vi "MatrixTest1.vi"() -> ()   [LabVIEW 2024]
uses:
  <vilib>/Analysis/baseanly.llb/Real A x B.vi
  <vilib>/Analysis/7linalg.llb/Real Transpose Matrix.vi
  <vilib>/Analysis/Matrix/Numeric/Conversions/Array To Matrix - RA.vi
  <vilib>/Analysis/Matrix/Numeric/Conversions/Matrix To Array - RM.vi
  <vilib>/Analysis/NI_AALBase.lvlib
  <vilib>/Analysis/Matrix/NI_Matrix.lvlib
  <vilib>/Analysis/NI_AALPro.lvlib
panel:
  in  "Array 11":i16[][](array[numeric])
  out "Array 8":i16[][](array[numeric])
  in  "Array 9":i16[][](array[numeric])
  out "Array 7":dbl[][](array[numeric])
  out "Array 6":dbl[][](array[numeric])
  in  "Array 5":i16[](array[numeric])
  in  "Array 4":i16[](array[numeric])
  out "x*y":dbl[](array[numeric])
  out "x+y":dbl[](array[numeric])
  out "Array 2":dbl[](array[numeric])
  out "Array 3":dbl[][](array[numeric])
  out "Array":dbl[](array[numeric])
  # "Conversion Matrix"
  # "Measured Data ( -> Sampling)"
  # "Resuls ( -> Sampling)"
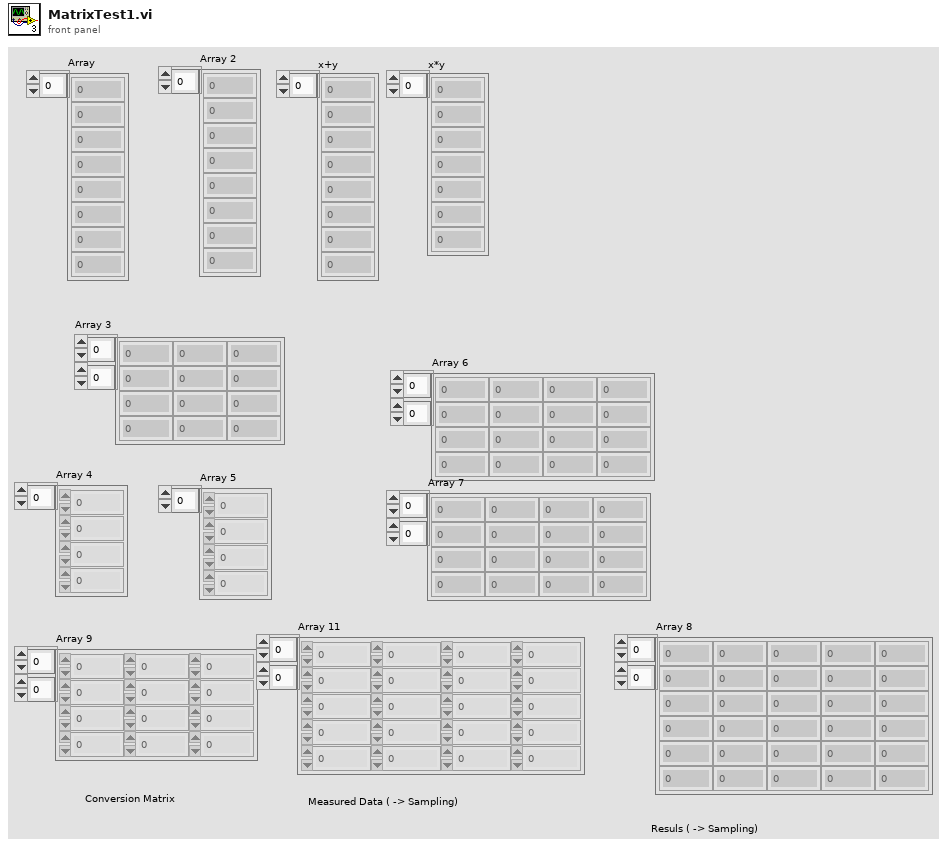
[diagram p1: front panel]
types:
  T1 = typedef "NI_Matrix.lvlib/RealMatrix.ctl" = dbl[][]
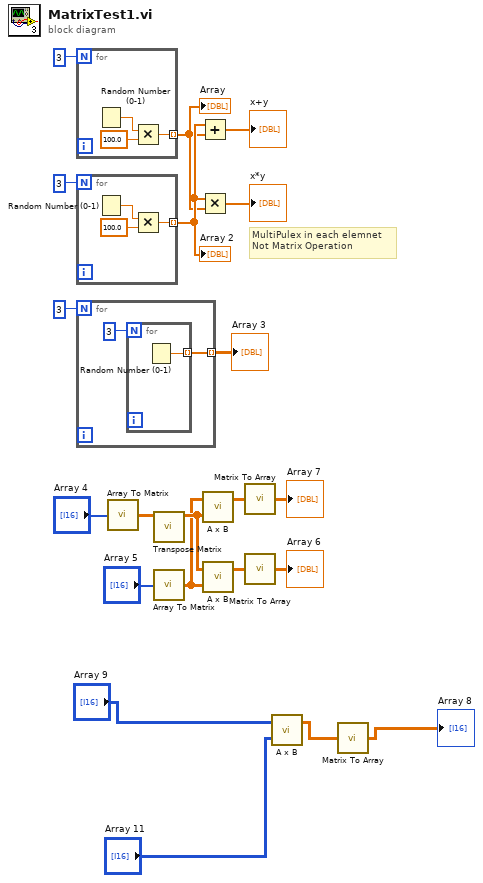
[diagram p0: block diagram]
diagram:
  # "MultiPulex in each elemnet\nNot Matrix Operation"
  n1 = for {
    N: 3 -> [_]
    tunnel: [w22] -> w15 mode=indexing
    n2 = Random Number (0-1)() -> (number: 0 to 1=w24:dbl)
    n3 = Multiply(x=w24, y=100.0) -> (x*y=w22:dbl)
  }
  "Array" <- w15
  n4 = for {
    N: 3 -> [_]
    tunnel: [w25] -> w16 mode=indexing
    n5 = Random Number (0-1)() -> (number: 0 to 1=w27:dbl)
    n6 = Multiply(x=w27, y=100.0) -> (x*y=w25:dbl)
  }
  "Array 2" <- w16
  n7 = for {
    N: 3 -> [_]
    tunnel: [w28] -> w19 mode=indexing
    n8 = for {
      N: 3 -> [_]
      tunnel: [w30] -> w28 mode=indexing
      n9 = Random Number (0-1)() -> (number: 0 to 1=w30:dbl)
    }
  }
  "Array 3" <- w19
  n10 = call-poly <vilib>:"Array To Matrix.vi"("Real 1D Array"="Array 4") -> ("Real Matrix (Column Vector)"=w9:T1)
  n11 = call-poly <vilib>:"Transpose Matrix.vi"("Input Matrix"=w9) -> ("Matrix Transpose"=w8:T1)  [unwired: 9 in, 1 out]
  n12 = call-poly <vilib>:"Array To Matrix.vi"("Real 1D Array"="Array 5") -> ("Real Matrix (Column Vector)"=w7:T1)
  n13 = Add(x=w16, y=w15) -> (x+y=→"x+y":dbl[])
  n14 = Multiply(x=w16, y=w15) -> (x*y=→"x*y":dbl[])
  n15 = call-poly <vilib>:"A x B.vi"("B"=w8, "A"=w7) -> ("A x B"=w6:T1)  [unwired: 1 out]
  n16 = call-poly <vilib>:"A x B.vi"("B"=w7, "A"=w8) -> ("A x B"=w11:T1)  [unwired: 1 out]
  n17 = call-poly <vilib>:"Matrix To Array.vi"("Real Matrix"=w6) -> ("Real 2D Array"=→"Array 7":dbl[][])
  n18 = call-poly <vilib>:"Matrix To Array.vi"("Real Matrix"=w11) -> ("Real 2D Array"=→"Array 6":dbl[][])
  n19 = call-poly <vilib>:"A x B.vi"("B"="Array 11", "A"="Array 9") -> ("A x B"=w4:T1)  [unwired: 1 out]
  n20 = call-poly <vilib>:"Matrix To Array.vi"("Real Matrix"=w4) -> ("Real 2D Array"=→"Array 8":dbl[][])
